vi "Steer_PD_Control.vi"(6 "Steering Kd":dbl(slide)=0.9985221674876847 scale=0.1..2.0 scale format="%#_2g", 9 "encoder counts":i32, 10 "Desired_Steer":dbl, 11 "Steering Kp":dbl) -> (2 "Vm":dbl, 3 "Steer":dbl)   [LabVIEW 2012]
uses:
  <vilib>/Simulation/Implementation/Shared/SIMSCR Execution Mode.ctl
  <vilib>/Simulation/Scripting/Companion Diagram/SimConfigNode/SimParams.ctl
  <vilib>/Simulation/Scripting/Companion Diagram/SimConfigNode/_simSolvers.ctl
  <vilib>/Simulation/Param Hierarchy/Typedefs/SIMPH Param Control Actions.ctl
  <vilib>/Simulation/Implementation/Shared/NILVSim_ParamChanged.vi
  <vilib>/Simulation/SignalArithmetic/Implementation/NILVSim Gain.llb/SIM Gain (scalar).vi
  <vilib>/Simulation/ContinuousLinear/Implementation/NILVSim Transfer Function Direct.llb/SIM Transfer Function Direct (SISO).vi
  <vilib>/Simulation/Nonlinear/Implementation/NILVSim Saturation.llb/SIM Saturation (scalar).vi
  <vilib>/Simulation/Implementation/Shared/NILVSim_Manager.vi
  <vilib>/Simulation/Implementation/Shared/NILVSim_FinalizeModel.vi
  <vilib>/Simulation/Implementation/Shared/SIM Unbundle Sim Info.vi
  <vilib>/Utility/error.llb/Clear Errors.vi
  <vilib>/Simulation/Implementation/Shared/NILVSim_GetModelError.vi
  <vilib>/Simulation/Implementation/Shared/SIM SimErrorHandler.vi
  <vilib>/Simulation/Implementation/Shared/SIM Bundle Sim Info.vi
  <vilib>/Simulation/Implementation/Shared/SIMSH Read Queue.vi
  <vilib>/Simulation/Implementation/Shared/NILVSim_Initialize.vi
  <vilib>/Simulation/Utility/Implementation/NILVSim Get Time and IsAcceptedStep.vi
  <vilib>/Simulation/Scripting/Companion Diagram/SimConfigNode/SimDog.xnode
  <vilib>/Simulation/Implementation/XNodeFramework/SimXNode/SimX.xnode
  <vilib>/Simulation/Implementation/Shared/NI_SIM_Implementation.lvlib
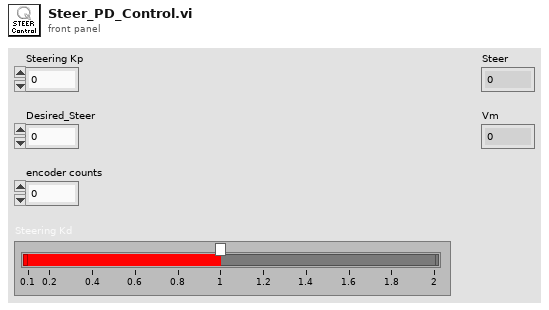
[diagram p1: front panel]
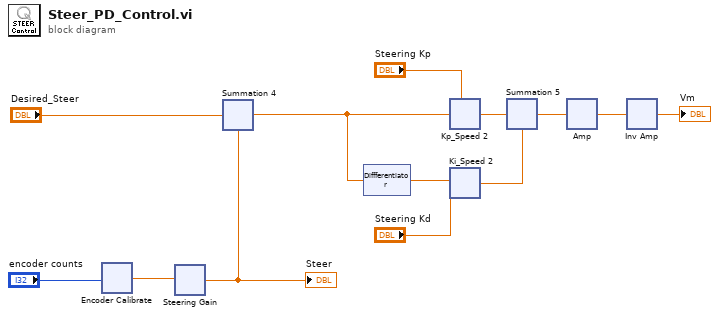
[diagram p0: block diagram]
diagram:
  n1 = xnode "Encoder Calibrate"("input"="encoder counts") -> ("output"=w2:dbl)  [unwired: 3 in]
  n2 = xnode "Steering Gain"("input"=w2) -> ("output"=w1:dbl)  [unwired: 3 in]
  "Steer" <- w1
  n3 = xnode ("Summation 4")("Operand1"="Desired_Steer", "Operand2"=w1) -> ("Result"=w9:dbl)
  n4 = xnode "Diffferentiator"("input u(k)"=w9) -> ("output y(k)"=w8:dbl)  [unwired: 4 in, 1 out]
  n5 = xnode ("Kp_Speed 2")("gain"="Steering Kp", "input"=w9) -> ("output"=w4:dbl)  [unwired: 2 in]
  n6 = xnode ("Ki_Speed 2")("gain"="Steering Kd", "input"=w8) -> ("output"=w5:dbl)  [unwired: 2 in]
  n7 = xnode ("Summation 5")("Operand1"=w4, "Operand2"=w5) -> ("Result"=w3:dbl)
  n8 = xnode "Amp"("input"=w3) -> ("output"=w7:dbl)  [unwired: 4 in]
  n9 = xnode "Inv Amp"("input"=w7) -> ("output"=→"Vm":dbl)  [unwired: 3 in]
